vi "Evaluate Loggable.vi"(6 "Level":T1, 11 "Application Log in":refnum<class "Application Log.lvclass">) -> (3 "Application Log out":refnum<class "Application Log.lvclass">, 4 "Log?":bool)   [LabVIEW 2016, in "Stream Log.lvlib" / "Application Log.lvclass"]
doc: "--\nCopyright © 2017 Composed SystemsI All rights reserved.\n\nAuthor: Jon McBee <jon.mcbee@composed.io>\n\nThis library is provided \"AS IS\" ,WITHOUT WARRANTIES OR\nCONDITIONS OF ANY KIND, either express or implied.\n\nComposed Systems -- composed.io\n\nStream 0.0.1.1\nJon McBee - Composed Systems\nCopyright (c) 2017, Composed Systems"
uses:
  <userlib>/Composed Systems/Stream/Log/Application Log/Application Log.lvclass
  <userlib>/Composed Systems/Stream/Log/Application Log/Log Level.ctl
  <userlib>/Composed Systems/Stream/Log/Application Log/Application Log.lvclass/Application Log.ctl
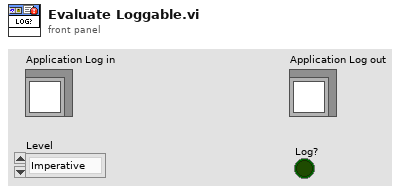
[diagram p1: front panel]
types:
  T1 = typedef "Stream Log.lvlib/Application Log.lvclass/Log Level.ctl" = enum16{"Imperative", "Major", "Minor", "Debug", "Off"}
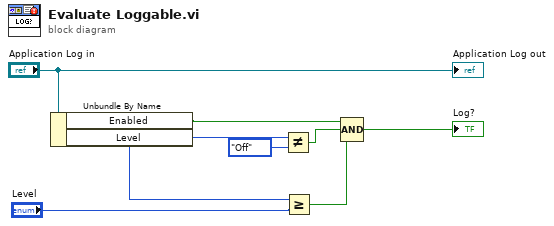
[diagram p0: block diagram]
diagram:
  n1 = Unbundle By Name("Application Log in") -> ("Enabled"=w1:bool, "Level"=w2:T1)
  n2 = Not Equal?(x=w2, y=Log_Level."Off") -> (x != y?=w5:bool)
  n3 = Greater Or Equal?(x=w2, y="Level") -> (x >= y?=w4:bool)
  n4 = Compound Arithmetic op=AND(w1, w5, w4) -> (→"Log?":bool)
  "Application Log out" <- "Application Log in"
